vi "Scan Setup Prep.vi"(8 "error in (no error)":errorcluster, 11 "Pulse Gen Scan in":refnum<class "Pulse Gen Scan.lvclass">) -> (0 "error out":errorcluster, 3 "Pulse Gen Scan out":refnum<class "Pulse Gen Scan.lvclass">)   [LabVIEW 2012, in "Pulse Gen Scan.lvclass"]
doc: "If in internal triggering mode, sets the overall period to 1 second to avoid conflicts when setting the new pattern. Also bundles the output on/off states into the Pulse Gen Scan object."
uses:
  Pulse Gen Scan.lvclass
  Pulse Gen Scan.lvclass/Pulse Gen Scan.ctl
  Global/GPIB Numbers.vi
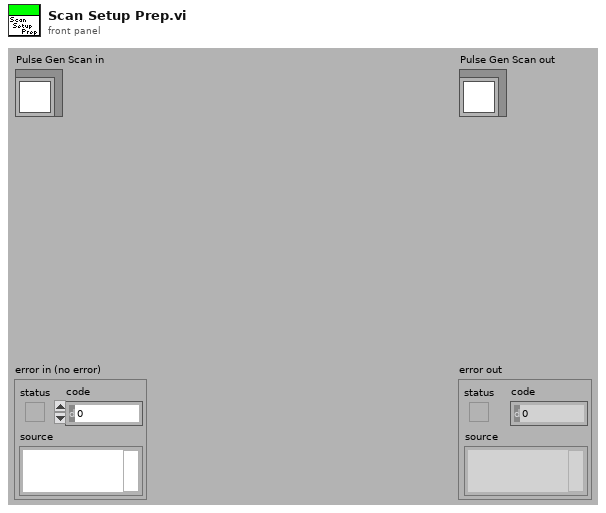
[diagram p1: front panel]
types:
  T1 = typedef "GPIB Type Def.ctl" = cluster{"Name":string, "bus":dbl, "GPIB":dbl, "GPIB as string":string, "byte":i32, "VISA Resource Name":refnum<visa-resource-name>}
  T2 = enum16{"Internal Oscillator", "Internal PLL", "Clock Input"}
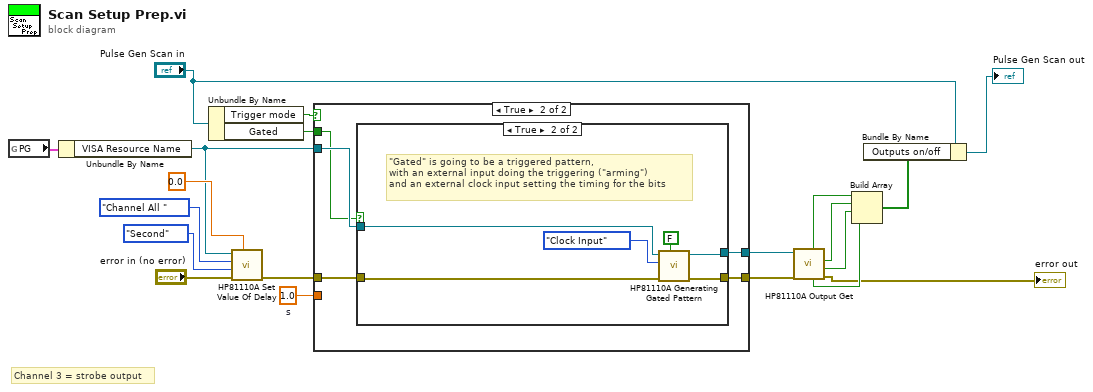
[diagram p0: block diagram]
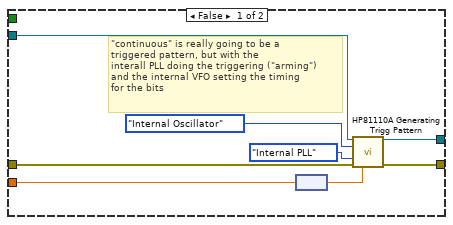
[diagram p2: hidden frame]
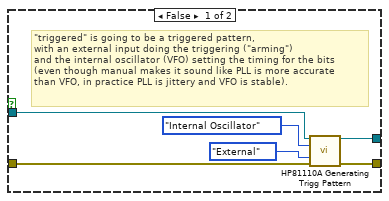
[diagram p3: hidden frame]
diagram:
  w13 = dbl[unit] 1.0  # s
  # "Channel 3 = strobe output"
  n1 = global read "GPIB Numbers.vi" "PG"() -> (w20:T1)
  n2 = Unbundle By Name(w20) -> ("VISA Resource Name"=w16:refnum<visa-resource-name>)
  n3 = Unbundle By Name("Pulse Gen Scan in") -> ("Trigger mode"=w2:bool, "Gated"=w1:bool)
  n4 = call "HP81110A Set Value Of Delay.vi"("Delay Value (0.0)"=0.0, "error in (no error)"="error in (no error)", "Delay Unit (0:Second)"=enum16{"Second", "Percent", "Degree", "Radians"}."Second", "Channel (1:Channel 1)"=enum16{"Channel All ", "Channel 1", "Channel 2"}."Channel All ", "VISA session"=w16) -> ("error out"=w15:errorcluster)  [unwired: 6 out]
  n5 = case shown="True" w2 {
    tunnel: w15 -> [w25 w32]
    tunnel: [w24 w31] -> w11
    tunnel: w16 -> [w26 w33]
    tunnel: w13 -> [w23 _]
    tunnel: [w21 w30] -> w12
    tunnel: w1 -> [_ w29]
    frame False {
      # "\"continuous\" is really going to be a \ntriggered pattern, but with the \ninterall PLL doing the triggering (\"arming\")\nand the internal VFO setting the timing \nfor the bits"
      n6 = node(w23) -> (w22:dbl)
      n7 = call "HP81110A Generating Trigg Pattern.vi"("VISA session"=w26, "Period Source (0:Internal Oscillator)"=T2."Internal Oscillator", "Trigger Source (0:Internal PLL)"=enum16{"Internal PLL", "External", "Manual"}."Internal PLL", "error in (no error)"=w25, "PLL Value (10.0E-6)"=w22) -> ("dup VISA session"=w21:refnum<visa-resource-name>, "error out"=w24:errorcluster)  [unwired: 3 in, 6 out]
    }
    frame True {
      n8 = case shown="True" w29 {
        tunnel: w33 -> [w38 w42]
        tunnel: w32 -> [w37 w40]
        tunnel: [w36 w44] -> w31
        tunnel: [w34 w43] -> w30
        frame False {
          # "\"triggered\" is going to be a triggered pattern, \nwith an external input doing the triggering (\"arming\")\nand the internal oscillator (VFO) setting the timing for the bits \n(even though manual makes it sound like PLL is more accurate \nthan VFO, in practice PLL is jittery and VFO is stable)."
          n9 = call "HP81110A Generating Trigg Pattern.vi"("VISA session"=w38, "Period Source (0:Internal Oscillator)"=T2."Internal Oscillator", "Trigger Source (0:Internal PLL)"=enum16{"Internal PLL", "External", "Manual"}."External", "error in (no error)"=w37) -> ("dup VISA session"=w34:refnum<visa-resource-name>, "error out"=w36:errorcluster)  [unwired: 4 in, 6 out]
        }
        frame True {
          # "\"Gated\" is going to be a triggered pattern, \nwith an external input doing the triggering (\"arming\")\nand an external clock input setting the timing for the bits"
          n10 = call "HP81110A Generating Gated Pattern.vi"("Gate Source (T:Manual)"=FALSE, "error in (no error)"=w40, "Period Source (0:Internal Oscillator)"=T2."Clock Input", "VISA session"=w42) -> ("error out"=w44:errorcluster, "dup VISA session"=w43:refnum<visa-resource-name>)  [unwired: 6 in]
        }
      }
    }
  }
  n11 = call "HP81110A Output Get.vi"("error in (no error)"=w11, "VISA session"=w12) -> ("error out"=→"error out":errorcluster, "output2OUT"=w8:bool, "notoutput1OUT"=w9:bool, "notoutput2OUT"=w7:bool, "output1OUT"=w10:bool)  [unwired: 4 in, 1 out]
  n12 = Build Array(w10, w9, w8, w7) -> (w4:bool[])
  n13 = Bundle By Name(cluster="Pulse Gen Scan in", "Outputs on/off"=w4) -> (→"Pulse Gen Scan out":refnum<class "Pulse Gen Scan.lvclass">)
